vi "Begin.vi"(11 "Image Size":T1=enum."320x240") -> (0 "error out":errorcluster)   [LabVIEW 2012]
doc: "Called before other user functions, this VI is expected to open initial I/O refnums, load in file data, and do all program initialization. Notice that the <B>error out</B> terminal is simply used for data flow. Wiring it to other structures or subVIs ensures that this VI runs first."
uses:
  <vilib>/Rock Robotics/WPI/Camera/WPI_CameraImageSize.ctl
  <vilib>/Rock Robotics/WPI/Camera/WPI_CameraWhite Balance Values.ctl
  <vilib>/Rock Robotics/WPI/Camera/WPI_CameraExposure Values.ctl
  <vilib>/Rock Robotics/WPI/Camera/WPI_CameraFrameRate.ctl
  <vilib>/Rock Robotics/WPI/DriverStation/WPI_DriverStationRobotMode2.ctl
  <vilib>/Rock Robotics/WPI/Joystick/WPI_JoystickDeviceEnum.ctl
  <vilib>/Rock Robotics/WPI/CAN/Jaguar/SubVIs/WPI_CANJaguar_ControlMode.ctl
  <vilib>/Rock Robotics/WPI/CAN/Jaguar/SubVIs/WPI_CANJaguar_PositionReference.ctl
  <vilib>/Rock Robotics/WPI/CAN/Jaguar/SubVIs/WPI_CANJaguar_SpeedReference.ctl
  <vilib>/Rock Robotics/SystemInterfaces/Typedef/FPGA_TypedefDigitalModule.ctl
  <vilib>/Rock Robotics/SystemInterfaces/DIO/FPGA_DIOPWMChannel.ctl
  <vilib>/Rock Robotics/SystemInterfaces/DIO/FPGA_DIOChannel.ctl
  <vilib>/Rock Robotics/SystemInterfaces/DIO/FPGA_DIORelayChannel.ctl
  <vilib>/Rock Robotics/WPI/Relay/WPI_RelayDirection.ctl
  Robot Global Data.vi
  <vilib>/Rock Robotics/WPI/MotorControl/WPI_MotorControlOpenCANJaguar.vi
  <vilib>/Rock Robotics/WPI/MotorControl/WPI_MotorControlOpen Victor.vi
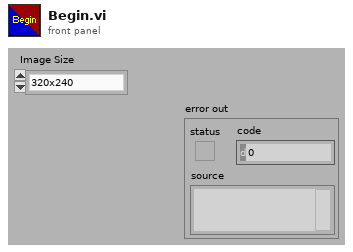
[diagram p1: front panel]
types:
  T1 = typedef "WPI_CameraImageSize.ctl" = enum16{"640x480", "320x240", "160x120"}
  T2 = typedef "WPI_RelayDirection.ctl" = enum16{"Both directions", "Forward only", "Reverse only"}
  T3 = typedef "FPGA_DIORelayChannel.ctl" = enum8{"Relay 1", "Relay 2", "Relay 3", "Relay 4", "Relay 5", "Relay 6", "Relay 7", "Relay 8", "Invalid"}
  T4 = typedef "FPGA_DIOChannel.ctl" = enum8{"DIO 1", "DIO 2", "DIO 3", "DIO 4", "DIO 5", "DIO 6", "DIO 7", "DIO 8", "DIO 9", "DIO 10", "DIO 11", "DIO 12", "DIO 13", "DIO 14", "Invalid"}
  T5 = typedef "FPGA_DIOPWMChannel.ctl" = enum8{"PWM 1", "PWM 2", "PWM 3", "PWM 4", "PWM 5", "PWM 6", "PWM 7", "PWM 8", "PWM 9", "PWM 10", "Invalid"}
  T6 = typedef "FPGA_TypedefDigitalModule.ctl" = enum16{"Digital Module 1", "Digital Module 2"}
  T7 = typedef "WPI_CANJaguar_SpeedReference.ctl" = u8
  T8 = typedef "WPI_CANJaguar_ControlMode.ctl" = enum8{"Percent VBus", "Current", "Speed", "Position", "Voltage"}
  T9 = typedef "WPI_CANJaguar_PositionReference.ctl" = u8
  T10 = typedef "WPI_JoystickDeviceEnum.ctl" = enum16{"USB 1", "USB 2", "USB 3", "USB 4", "Kinect 1", "Kinect 2"}
  T11 = typedef "WPI_DriverStationRobotMode2.ctl" = enum16{"Autonomous Disabled", "Autonomous Enabled", "Teleop Disabled", "Teleop Enabled", "Timeout", "Finish", "Test Disabled", "Test Enabled"}
  T12 = typedef "WPI_CameraFrameRate.ctl" = u32
  T13 = typedef "WPI_CameraExposure Values.ctl" = enum16{"Auto", "Flicker-free 50 Hz", "Flicker-free 60 Hz", "Hold current"}
  T14 = typedef "WPI_CameraWhite Balance Values.ctl" = enum16{"Auto", "Fixed indoor", "Fixed outdoor 1", "Fixed outdoor 2", "Fixed fluorescent 1", "Fixed fluorescent 2", "Hold current"}
  T15 = typedef "WPI_JoystickDevRef.ctl" = cluster{"Device":T10}
  T16 = typedef "WPI_CameraDevRef.ctl" = cluster{"Camera Address":string, "CameraStatus":errorcluster, "Acquire Image Notifier":refnum<notifier>}
  T17 = typedef "WPI_MotorControlDeviceRef.ctl" = cluster{"DeviceStatus":errorcluster, "Type":enum16{"PWM", "CAN"}, "PWM":cluster{"Digital Module":T6, "PWM Channel":T5, "DeadBand":T18}, "CAN":cluster{"Device Number":u8, "Control Mode":T8, "Semaphore":T19, "Max Vout":dbl}, "Invert":bool, "TransformRef":T20, "InvTransformRef":T20}
  T18 = typedef "WPI_PWMDeadband.ctl" = cluster{"Name":string, "maxPositivePwm":i32, "minPositivePwm":i32, "centerPwm":i32, "maxNegativePwm":i32, "minNegativePwm":i32, "angularRange":u16}
  T19 = typedef "Semaphore RefNum" = refnum<k1>
  T20 = typedef "WPI_PWMTransform_ConPane.ctl" = refnum<vi>
  T21 = typedef "WPI_DigitalInputDevRef.ctl" = cluster{"DevStatus":errorcluster, "DIO Channel":T4, "Digital Module":T6}
  T22 = typedef "WPI_RelayDevRef.ctl" = cluster{"DevStatus":errorcluster, "Relay Channel":T3, "Digital Module":T6, "Relay Direction":T2}
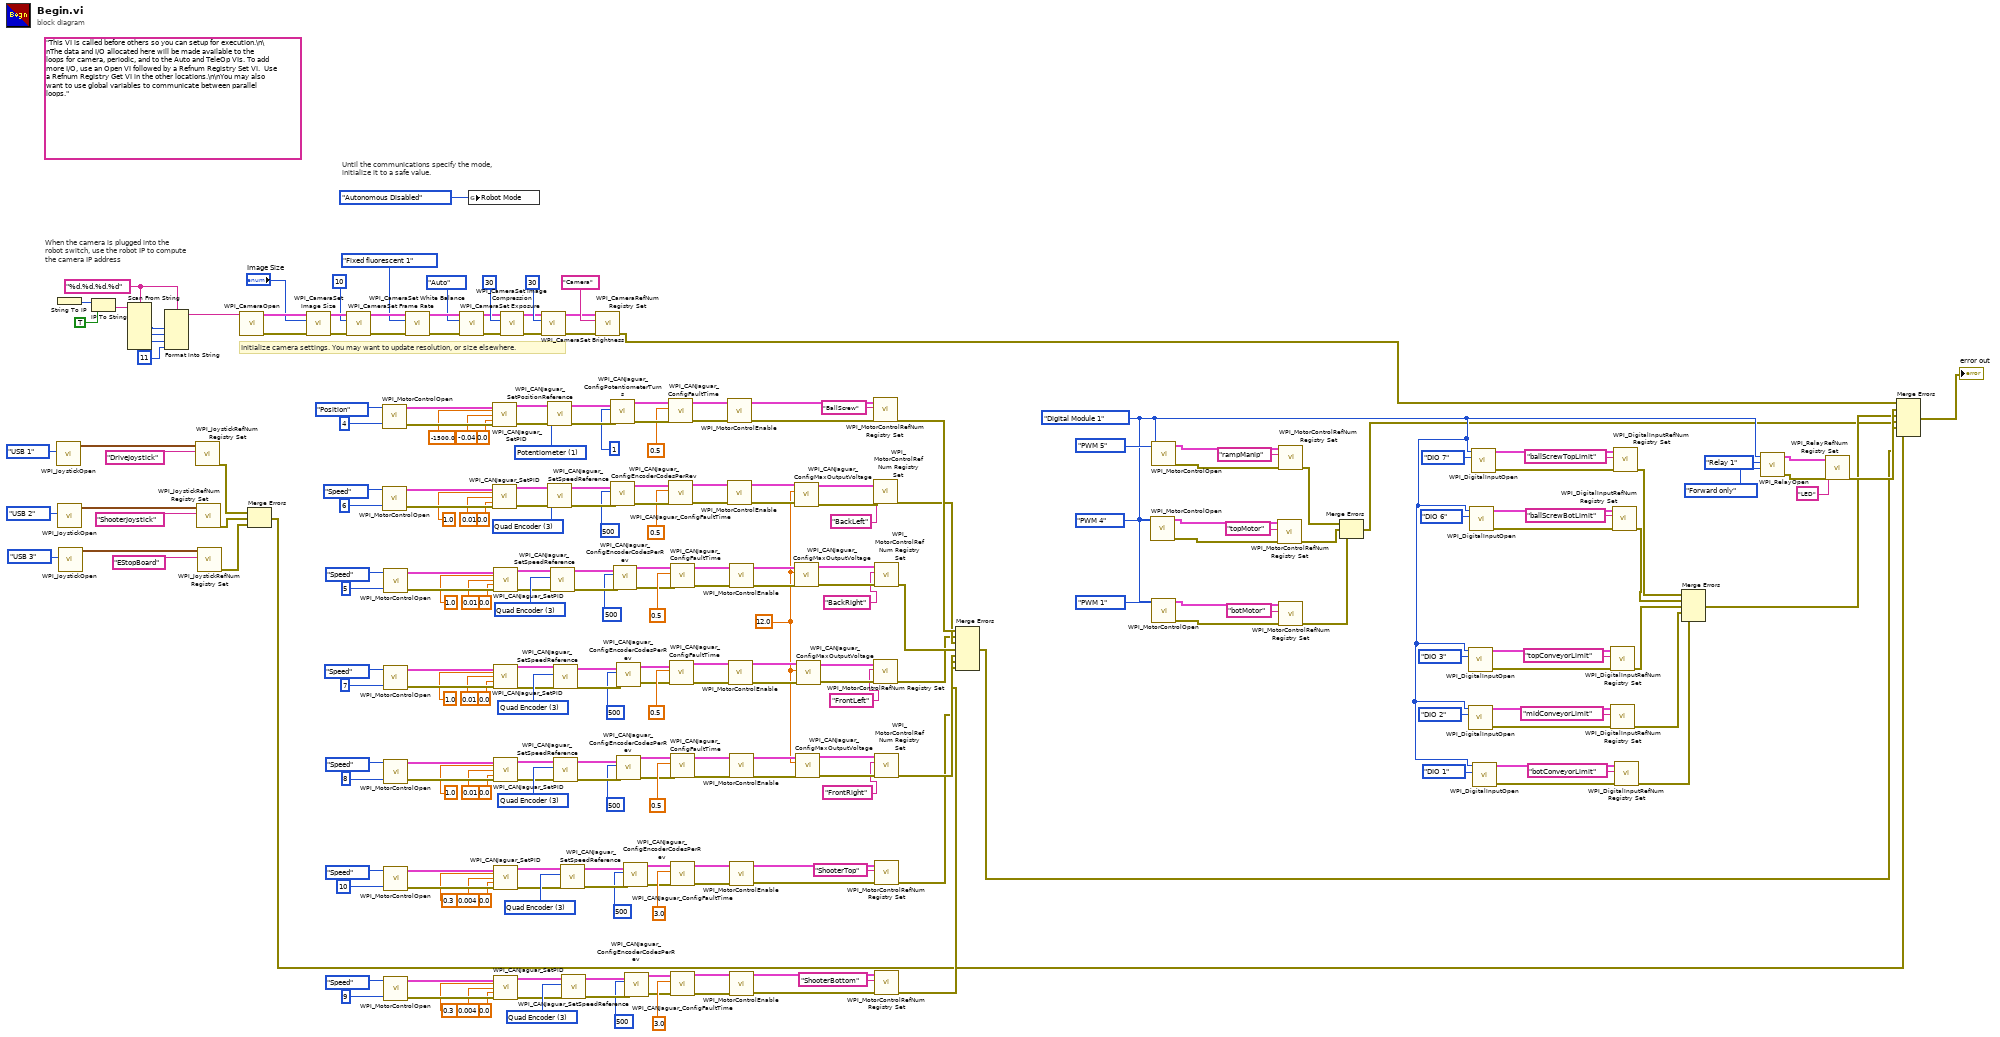
[diagram p0: block diagram]
diagram:
  w11 = FPGA_TypedefDigitalModule."Digital Module 1" ("Digital Module (Module 1)")
  w86 = T7 3 items=["Encoder"=0, "Inv Encoder"=2, "Quad Encoder"=3, "None"=255] ("Speed Reference")
  w90 = T7 3 items=["Encoder"=0, "Inv Encoder"=2, "Quad Encoder"=3, "None"=255] ("Speed Reference")
  w94 = T7 3 items=["Encoder"=0, "Inv Encoder"=2, "Quad Encoder"=3, "None"=255] ("Speed Reference")
  w98 = T7 3 items=["Encoder"=0, "Inv Encoder"=2, "Quad Encoder"=3, "None"=255] ("Speed Reference")
  w102 = T7 3 items=["Encoder"=0, "Inv Encoder"=2, "Quad Encoder"=3, "None"=255] ("Speed Reference")
  w106 = 12.0 ("Fault Time (s)")
  w127 = T7 3 items=["Encoder"=0, "Inv Encoder"=2, "Quad Encoder"=3, "None"=255] ("Speed Reference")
  w210 = T9 1 items=["Quad Encoder"=0, "Potentiometer"=1, "None"=255] ("Position Reference")
  w231 = "%d.%d.%d.%d" ("format string")
  (unwired) "This VI is called before others so you can setup for execution.\n\nThe data and I/O allocated here will be made available to the loops for camera, periodic, and to the Auto and TeleOp VIs. To add more I/O, use an Open VI followed by a Refnum Registry Set VI.  Use a Refnum Registry Get VI in the other locations.\n\nYou may also want to use global variables to communicate between parallel loops."
  # "Until the communications specify the mode,\ninitialize it to a safe value."
  # "When the camera is plugged into the\nrobot switch, use the robot IP to compute\nthe camera IP address"
  # "Initialize camera settings. You may want to update resolution, or size elsewhere."
  n1 = call <vilib>:"WPI_JoystickOpen.vi"("JoystickDevice"=WPI_JoystickDeviceEnum."USB 1") -> ("JoystickDevRef"=w227:T15)  [unwired: 10 in]
  n2 = String To IP() -> (0:w238:u32)  [unwired: 1 in]
  n3 = call <vilib>:"WPI_JoystickOpen.vi"("JoystickDevice"=WPI_JoystickDeviceEnum."USB 2") -> ("JoystickDevRef"=w224:T15)  [unwired: 10 in]
  n4 = call <vilib>:"WPI_JoystickOpen.vi"("JoystickDevice"=WPI_JoystickDeviceEnum."USB 3") -> ("JoystickDevRef"=w221:T15)  [unwired: 10 in]
  n5 = IP To String(1:TRUE ("dot notation? (F)"), 2:w238) -> (0:w236:string)
  n6 = Scan From String(format string=w231, input string=w236) -> (output 1=w235:i32, output 2=w234:i32, output 3=w233:i32)  [unwired: 7 in, 3 out]
  n7 = Format Into String(format string=w231, w235, w234, w233, 11 ("Compression")) -> (resulting string=w229:string)  [unwired: 2 in, 1 out]
  n8 = call <vilib>:"WPI_JoystickRefNum Registry Set.vi"("refnum name"="DriveJoystick", "JoystickDevRef"=w227) -> ("error out"=w63:errorcluster)  [unwired: 8 in, 1 out]
  n9 = call <vilib>:"WPI_JoystickRefNum Registry Set.vi"("refnum name"="ShooterJoystick", "JoystickDevRef"=w224) -> ("error out"=w62:errorcluster)  [unwired: 8 in, 1 out]
  n10 = call <vilib>:"WPI_JoystickRefNum Registry Set.vi"("refnum name"="EStopBoard", "JoystickDevRef"=w221) -> ("error out"=w61:errorcluster)  [unwired: 8 in, 1 out]
  n11 = call <vilib>:"WPI_CameraOpen.vi"("Camera Address"=w229) -> ("error out"=w250:errorcluster, "CameraDevRef"=w251:T16)  [unwired: 1 in, 8 out]
  n12 = Merge Errors(w63, w62, w61) -> (w2:errorcluster)
  n13 = call <vilib>:"WPI_CameraSet Image Size.vi"("error in (no error)"=w250, "Image Size"="Image Size", "CameraDevRef"=w251) -> ("error out"=w249:errorcluster, "CameraDevRef Out"=w252:T16)  [unwired: 7 out]
  n14 = call <vilib>:"WPI_CameraSet Frame Rate.vi"("error in (no error)"=w249, "Frame Rate (fps)"=T12 10, "CameraDevRef"=w252) -> ("error out"=w248:errorcluster, "CameraDevRef Out"=w254:T16)  [unwired: 7 out]
  n15 = call-poly <vilib>:"WPI_MotorControlOpen.vi"("Device Number"=u8 4, "Control Mode"=WPI_CANJaguar_ControlMode."Position") -> ("error out"=w216:errorcluster, "MotorControlDeviceRef"=w217:T17)  [unwired: 8 in]
  n16 = call-poly <vilib>:"WPI_MotorControlOpen.vi"("Device Number"=u8 6, "Control Mode"=WPI_CANJaguar_ControlMode."Speed") -> ("error out"=w196:errorcluster, "MotorControlDeviceRef"=w197:T17)  [unwired: 8 in]
  n17 = call-poly <vilib>:"WPI_MotorControlOpen.vi"("Device Number"=u8 7, "Control Mode"=WPI_CANJaguar_ControlMode."Speed") -> ("error out"=w169:errorcluster, "MotorControlDeviceRef"=w170:T17)  [unwired: 8 in]
  n18 = call-poly <vilib>:"WPI_MotorControlOpen.vi"("Device Number"=u8 5, "Control Mode"=WPI_CANJaguar_ControlMode."Speed") -> ("error out"=w179:errorcluster, "MotorControlDeviceRef"=w180:T17)  [unwired: 8 in]
  n19 = call-poly <vilib>:"WPI_MotorControlOpen.vi"("Device Number"=u8 8, "Control Mode"=WPI_CANJaguar_ControlMode."Speed") -> ("error out"=w159:errorcluster, "MotorControlDeviceRef"=w160:T17)  [unwired: 8 in]
  n20 = call-poly <vilib>:"WPI_MotorControlOpen.vi"("Device Number"=u8 10, "Control Mode"=WPI_CANJaguar_ControlMode."Speed") -> ("error out"=w149:errorcluster, "MotorControlDeviceRef"=w150:T17)  [unwired: 8 in]
  n21 = call-poly <vilib>:"WPI_MotorControlOpen.vi"("Device Number"=u8 9, "Control Mode"=WPI_CANJaguar_ControlMode."Speed") -> ("error out"=w137:errorcluster, "MotorControlDeviceRef"=w138:T17)  [unwired: 8 in]
  n22 = call <vilib>:"WPI_CameraSet White Balance.vi"("error in (no error)"=w248, "White Balance"=WPI_CameraWhite_Balance_Values."Fixed fluorescent 1", "CameraDevRef"=w254) -> ("error out"=w247:errorcluster, "CameraDevRef Out"=w253:T16)  [unwired: 7 out]
  n23 = call <vilib>:"WPI_CameraSet Exposure.vi"("error in (no error)"=w247, "Exposure"=WPI_CameraExposure_Values."Auto", "CameraDevRef"=w253) -> ("error out"=w246:errorcluster, "CameraDevRef Out"=w256:T16)  [unwired: 7 out]
  n24 = global write "Robot Global Data.vi" "Robot Mode"(WPI_DriverStationRobotMode2."Autonomous Disabled" ("Robot Mode")) -> ()
  n25 = call <vilib>:"WPI_CANJaguar_SetPID.vi"("CAN Jaguar Ref"=w217, "P"=-1500.0, "I"=-0.04, "D"=0.0, "error in (no error)"=w216) -> ("CAN Jaguar Ref Out"=w212:T17, "error out"=w211:errorcluster)  [unwired: 9 in]
  n26 = call <vilib>:"WPI_CANJaguar_SetPID.vi"("CAN Jaguar Ref"=w197, "P"=1.0, "I"=0.01, "D"=0.0, "error in (no error)"=w196) -> ("CAN Jaguar Ref Out"=w192:T17, "error out"=w191:errorcluster)  [unwired: 9 in]
  n27 = call <vilib>:"WPI_CANJaguar_SetPID.vi"("CAN Jaguar Ref"=w170, "P"=1.0, "I"=0.01, "D"=0.0, "error in (no error)"=w169) -> ("CAN Jaguar Ref Out"=w69:T17, "error out"=w68:errorcluster)  [unwired: 9 in]
  n28 = call <vilib>:"WPI_CANJaguar_SetPID.vi"("CAN Jaguar Ref"=w180, "P"=1.0, "I"=0.01, "D"=0.0, "error in (no error)"=w179) -> ("CAN Jaguar Ref Out"=w73:T17, "error out"=w72:errorcluster)  [unwired: 9 in]
  n29 = call <vilib>:"WPI_CANJaguar_SetPID.vi"("CAN Jaguar Ref"=w160, "P"=1.0, "I"=0.01, "D"=0.0, "error in (no error)"=w159) -> ("CAN Jaguar Ref Out"=w76:T17, "error out"=w77:errorcluster)  [unwired: 9 in]
  n30 = call <vilib>:"WPI_CANJaguar_SetPID.vi"("CAN Jaguar Ref"=w150, "P"=0.3, "I"=0.004, "D"=0.0, "error in (no error)"=w149) -> ("CAN Jaguar Ref Out"=w78:T17, "error out"=w79:errorcluster)  [unwired: 9 in]
  n31 = call <vilib>:"WPI_CANJaguar_SetPID.vi"("CAN Jaguar Ref"=w138, "P"=0.3, "I"=0.004, "D"=0.0, "error in (no error)"=w137) -> ("CAN Jaguar Ref Out"=w85:T17, "error out"=w84:errorcluster)  [unwired: 9 in]
  n32 = call <vilib>:"WPI_CameraSet Image Compression.vi"("error in (no error)"=w246, "Compression"=30, "CameraDevRef"=w256) -> ("error out"=w245:errorcluster, "CameraDevRef Out"=w255:T16)  [unwired: 7 out]
  n33 = call <vilib>:"WPI_CameraSet Brightness.vi"("error in (no error)"=w245, "Brightness"=30, "CameraDevRef"=w255) -> ("error out"=w243:errorcluster, "CameraDevRef Out"=w244:T16)  [unwired: 7 out]
  n34 = call <vilib>:"WPI_CANJaguar_SetPositionReference.vi"("error in (no error)"=w211, "Position Reference"=w210, "CAN Jaguar Ref"=w212) -> ("error out"=w208:errorcluster, "CAN Jaguar Ref Out"=w209:T17)  [unwired: 7 in]
  n35 = call <vilib>:"WPI_CANJaguar_SetSpeedReference.vi"("error in (no error)"=w191, "Speed Reference"=w127, "CAN Jaguar Ref"=w192) -> ("error out"=w189:errorcluster, "CAN Jaguar Ref Out"=w190:T17)  [unwired: 7 in]
  n36 = call <vilib>:"WPI_CANJaguar_SetSpeedReference.vi"("error in (no error)"=w72, "Speed Reference"=w102, "CAN Jaguar Ref"=w73) -> ("error out"=w104:errorcluster, "CAN Jaguar Ref Out"=w105:T17)  [unwired: 7 in]
  n37 = call <vilib>:"WPI_CANJaguar_SetSpeedReference.vi"("error in (no error)"=w68, "Speed Reference"=w98, "CAN Jaguar Ref"=w69) -> ("error out"=w100:errorcluster, "CAN Jaguar Ref Out"=w101:T17)  [unwired: 7 in]
  n38 = call <vilib>:"WPI_CANJaguar_SetSpeedReference.vi"("error in (no error)"=w77, "Speed Reference"=w94, "CAN Jaguar Ref"=w76) -> ("error out"=w96:errorcluster, "CAN Jaguar Ref Out"=w97:T17)  [unwired: 7 in]
  n39 = call <vilib>:"WPI_CANJaguar_SetSpeedReference.vi"("error in (no error)"=w79, "Speed Reference"=w90, "CAN Jaguar Ref"=w78) -> ("error out"=w92:errorcluster, "CAN Jaguar Ref Out"=w93:T17)  [unwired: 7 in]
  n40 = call <vilib>:"WPI_CANJaguar_SetSpeedReference.vi"("error in (no error)"=w84, "Speed Reference"=w86, "CAN Jaguar Ref"=w85) -> ("error out"=w88:errorcluster, "CAN Jaguar Ref Out"=w89:T17)  [unwired: 7 in]
  n41 = call <vilib>:"WPI_CameraRefNum Registry Set.vi"("error in (no error)"=w243, "refnum name"="Camera", "CameraDevRef"=w244) -> ("error out"=w1:errorcluster)  [unwired: 8 out]
  n42 = call <vilib>:"WPI_CANJaguar_ConfigPotentiometerTurns.vi"("error in (no error)"=w208, "Potentiometer Turns"=u16 1, "CAN Jaguar Ref"=w209) -> ("error out"=w205:errorcluster, "CAN Jaguar Ref Out"=w206:T17)  [unwired: 7 in]
  n43 = call <vilib>:"WPI_CANJaguar_ConfigEncoderCodesPerRev.vi"("error in (no error)"=w189, "Encoder Codes Per Rev"=u16 500 ("Potentiometer Turns"), "CAN Jaguar Ref"=w190) -> ("error out"=w186:errorcluster, "CAN Jaguar Ref Out"=w187:T17)  [unwired: 7 in]
  n44 = call <vilib>:"WPI_CANJaguar_ConfigEncoderCodesPerRev.vi"("error in (no error)"=w104, "Encoder Codes Per Rev"=u16 500 ("Potentiometer Turns"), "CAN Jaguar Ref"=w105) -> ("error out"=w71:errorcluster, "CAN Jaguar Ref Out"=w70:T17)  [unwired: 7 in]
  n45 = call <vilib>:"WPI_CANJaguar_ConfigEncoderCodesPerRev.vi"("error in (no error)"=w100, "Encoder Codes Per Rev"=u16 500 ("Potentiometer Turns"), "CAN Jaguar Ref"=w101) -> ("error out"=w66:errorcluster, "CAN Jaguar Ref Out"=w67:T17)  [unwired: 7 in]
  n46 = call <vilib>:"WPI_CANJaguar_ConfigEncoderCodesPerRev.vi"("error in (no error)"=w96, "Encoder Codes Per Rev"=u16 500 ("Potentiometer Turns"), "CAN Jaguar Ref"=w97) -> ("error out"=w75:errorcluster, "CAN Jaguar Ref Out"=w74:T17)  [unwired: 7 in]
  n47 = call <vilib>:"WPI_CANJaguar_ConfigEncoderCodesPerRev.vi"("error in (no error)"=w92, "Encoder Codes Per Rev"=u16 500 ("Potentiometer Turns"), "CAN Jaguar Ref"=w93) -> ("error out"=w81:errorcluster, "CAN Jaguar Ref Out"=w80:T17)  [unwired: 7 in]
  n48 = call <vilib>:"WPI_CANJaguar_ConfigEncoderCodesPerRev.vi"("error in (no error)"=w88, "Encoder Codes Per Rev"=u16 500 ("Potentiometer Turns"), "CAN Jaguar Ref"=w89) -> ("error out"=w82:errorcluster, "CAN Jaguar Ref Out"=w83:T17)  [unwired: 7 in]
  n49 = call <vilib>:"WPI_CANJaguar_ConfigFaultTime.vi"("error in (no error)"=w205, "Fault Time (s)"=0.5, "CAN Jaguar Ref"=w206) -> ("error out"=w202:errorcluster, "CAN Jaguar Ref Out"=w203:T17)  [unwired: 7 in]
  n50 = call <vilib>:"WPI_CANJaguar_ConfigFaultTime.vi"("error in (no error)"=w186, "Fault Time (s)"=0.5, "CAN Jaguar Ref"=w187) -> ("error out"=w183:errorcluster, "CAN Jaguar Ref Out"=w184:T17)  [unwired: 7 in]
  n51 = call <vilib>:"WPI_CANJaguar_ConfigFaultTime.vi"("error in (no error)"=w66, "Fault Time (s)"=0.5, "CAN Jaguar Ref"=w67) -> ("error out"=w163:errorcluster, "CAN Jaguar Ref Out"=w164:T17)  [unwired: 7 in]
  n52 = call <vilib>:"WPI_CANJaguar_ConfigFaultTime.vi"("error in (no error)"=w71, "Fault Time (s)"=0.5, "CAN Jaguar Ref"=w70) -> ("error out"=w173:errorcluster, "CAN Jaguar Ref Out"=w174:T17)  [unwired: 7 in]
  n53 = call <vilib>:"WPI_CANJaguar_ConfigFaultTime.vi"("error in (no error)"=w75, "Fault Time (s)"=0.5, "CAN Jaguar Ref"=w74) -> ("error out"=w153:errorcluster, "CAN Jaguar Ref Out"=w154:T17)  [unwired: 7 in]
  n54 = call <vilib>:"WPI_CANJaguar_ConfigFaultTime.vi"("error in (no error)"=w81, "Fault Time (s)"=3.0, "CAN Jaguar Ref"=w80) -> ("error out"=w143:errorcluster, "CAN Jaguar Ref Out"=w144:T17)  [unwired: 7 in]
  n55 = call <vilib>:"WPI_CANJaguar_ConfigFaultTime.vi"("error in (no error)"=w82, "Fault Time (s)"=3.0, "CAN Jaguar Ref"=w83) -> ("error out"=w131:errorcluster, "CAN Jaguar Ref Out"=w132:T17)  [unwired: 7 in]
  n56 = call <vilib>:"WPI_MotorControlEnable.vi"("error in (no error)"=w202, "CAN Jaguar Ref"=w203) -> ("error out"=w200:errorcluster, "CAN Jaguar Ref Out"=w201:T17)  [unwired: 8 in]
  n57 = call <vilib>:"WPI_MotorControlEnable.vi"("error in (no error)"=w183, "CAN Jaguar Ref"=w184) -> ("error out"=w125:errorcluster, "CAN Jaguar Ref Out"=w126:T17)  [unwired: 8 in]
  n58 = call <vilib>:"WPI_MotorControlEnable.vi"("error in (no error)"=w163, "CAN Jaguar Ref"=w164) -> ("error out"=w113:errorcluster, "CAN Jaguar Ref Out"=w114:T17)  [unwired: 8 in]
  n59 = call <vilib>:"WPI_MotorControlEnable.vi"("error in (no error)"=w173, "CAN Jaguar Ref"=w174) -> ("error out"=w120:errorcluster, "CAN Jaguar Ref Out"=w121:T17)  [unwired: 8 in]
  n60 = call <vilib>:"WPI_MotorControlEnable.vi"("error in (no error)"=w153, "CAN Jaguar Ref"=w154) -> ("error out"=w110:errorcluster, "CAN Jaguar Ref Out"=w111:T17)  [unwired: 8 in]
  n61 = call <vilib>:"WPI_MotorControlEnable.vi"("error in (no error)"=w143, "CAN Jaguar Ref"=w144) -> ("error out"=w141:errorcluster, "CAN Jaguar Ref Out"=w142:T17)  [unwired: 8 in]
  n62 = call <vilib>:"WPI_MotorControlEnable.vi"("error in (no error)"=w131, "CAN Jaguar Ref"=w132) -> ("error out"=w129:errorcluster, "CAN Jaguar Ref Out"=w130:T17)  [unwired: 8 in]
  n63 = call <vilib>:"WPI_CANJaguar_ConfigMaxOutputVoltage.vi"("error in (no error)"=w120, "Maximum Output Voltage"=w106, "CAN Jaguar Ref"=w121) -> ("error out"=w119:errorcluster, "CAN Jaguar Ref Out"=w118:T17)  [unwired: 7 in]
  n64 = call <vilib>:"WPI_CANJaguar_ConfigMaxOutputVoltage.vi"("error in (no error)"=w125, "Maximum Output Voltage"=w106, "CAN Jaguar Ref"=w126) -> ("error out"=w124:errorcluster, "CAN Jaguar Ref Out"=w123:T17)  [unwired: 7 in]
  n65 = call <vilib>:"WPI_CANJaguar_ConfigMaxOutputVoltage.vi"("error in (no error)"=w110, "Maximum Output Voltage"=w106, "CAN Jaguar Ref"=w111) -> ("error out"=w108:errorcluster, "CAN Jaguar Ref Out"=w109:T17)  [unwired: 7 in]
  n66 = call <vilib>:"WPI_CANJaguar_ConfigMaxOutputVoltage.vi"("error in (no error)"=w113, "Maximum Output Voltage"=w106, "CAN Jaguar Ref"=w114) -> ("error out"=w115:errorcluster, "CAN Jaguar Ref Out"=w116:T17)  [unwired: 7 in]
  n67 = call <vilib>:"WPI_MotorControlRefNum Registry Set.vi"("error in (no error)"=w200, "refnum name"="BallScrew", "MotorControlDevRef"=w201) -> ("error out"=w60:errorcluster)  [unwired: 7 in, 1 out]
  n68 = call <vilib>:"WPI_MotorControlRefNum Registry Set.vi"("error in (no error)"=w124, "refnum name"="BackLeft", "MotorControlDevRef"=w123) -> ("error out"=w59:errorcluster)  [unwired: 7 in, 1 out]
  n69 = call <vilib>:"WPI_MotorControlRefNum Registry Set.vi"("error in (no error)"=w115, "refnum name"="FrontLeft", "MotorControlDevRef"=w116) -> ("error out"=w57:errorcluster)  [unwired: 7 in, 1 out]
  n70 = call <vilib>:"WPI_MotorControlRefNum Registry Set.vi"("error in (no error)"=w119, "refnum name"="BackRight", "MotorControlDevRef"=w118) -> ("error out"=w58:errorcluster)  [unwired: 7 in, 1 out]
  n71 = call <vilib>:"WPI_MotorControlRefNum Registry Set.vi"("error in (no error)"=w108, "refnum name"="FrontRight", "MotorControlDevRef"=w109) -> ("error out"=w56:errorcluster)  [unwired: 7 in, 1 out]
  n72 = call <vilib>:"WPI_MotorControlRefNum Registry Set.vi"("error in (no error)"=w141, "refnum name"="ShooterTop", "MotorControlDevRef"=w142) -> ("error out"=w55:errorcluster)  [unwired: 7 in, 1 out]
  n73 = call <vilib>:"WPI_MotorControlRefNum Registry Set.vi"("error in (no error)"=w129, "refnum name"="ShooterBottom", "MotorControlDevRef"=w130) -> ("error out"=w54:errorcluster)  [unwired: 7 in, 1 out]
  n74 = Merge Errors(w60, w57, w59, w58, w56, w55, w54) -> (w3:errorcluster)
  n75 = call-poly <vilib>:"WPI_MotorControlOpen.vi"("PWM Channel"=FPGA_DIOPWMChannel."PWM 4", "Digital Module (Module 1)"=w11) -> ("error out"=w46:errorcluster, "MotorControlDeviceRef"=w48:T17)  [unwired: 8 in]
  n76 = call-poly <vilib>:"WPI_MotorControlOpen.vi"("PWM Channel"=FPGA_DIOPWMChannel."PWM 5", "Digital Module (Module 1)"=w11) -> ("error out"=w50:errorcluster, "MotorControlDeviceRef"=w52:T17)  [unwired: 8 in]
  n77 = call-poly <vilib>:"WPI_MotorControlOpen.vi"("PWM Channel"=FPGA_DIOPWMChannel."PWM 1", "Digital Module (Module 1)"=w11) -> ("error out"=w42:errorcluster, "MotorControlDeviceRef"=w44:T17)  [unwired: 8 in]
  n78 = call <vilib>:"WPI_MotorControlRefNum Registry Set.vi"("error in (no error)"=w46, "refnum name"="topMotor", "MotorControlDevRef"=w48) -> ("error out"=w40:errorcluster)  [unwired: 7 in, 1 out]
  n79 = call <vilib>:"WPI_MotorControlRefNum Registry Set.vi"("error in (no error)"=w50, "refnum name"="rampManip", "MotorControlDevRef"=w52) -> ("error out"=w41:errorcluster)  [unwired: 7 in, 1 out]
  n80 = call <vilib>:"WPI_MotorControlRefNum Registry Set.vi"("error in (no error)"=w42, "refnum name"="botMotor", "MotorControlDevRef"=w44) -> ("error out"=w39:errorcluster)  [unwired: 7 in, 1 out]
  n81 = Merge Errors(w41, w40, w39) -> (w4:errorcluster)
  n82 = call <vilib>:"WPI_DigitalInputOpen.vi"("DIO Channel"=FPGA_DIOChannel."DIO 3", "Digital Module (Module 1)"=w11) -> ("error out"=w28:errorcluster, "DigitalInputDevRef"=w29:T21)  [unwired: 8 in]
  n83 = call <vilib>:"WPI_DigitalInputOpen.vi"("DIO Channel"=FPGA_DIOChannel."DIO 2", "Digital Module (Module 1)"=w11) -> ("error out"=w24:errorcluster, "DigitalInputDevRef"=w25:T21)  [unwired: 8 in]
  n84 = call <vilib>:"WPI_DigitalInputOpen.vi"("DIO Channel"=FPGA_DIOChannel."DIO 6", "Digital Module (Module 1)"=w11) -> ("error out"=w32:errorcluster, "DigitalInputDevRef"=w33:T21)  [unwired: 8 in]
  n85 = call <vilib>:"WPI_DigitalInputOpen.vi"("DIO Channel"=FPGA_DIOChannel."DIO 7", "Digital Module (Module 1)"=w11) -> ("error out"=w36:errorcluster, "DigitalInputDevRef"=w37:T21)  [unwired: 8 in]
  n86 = call <vilib>:"WPI_DigitalInputOpen.vi"("DIO Channel"=FPGA_DIOChannel."DIO 1", "Digital Module (Module 1)"=w11) -> ("error out"=w20:errorcluster, "DigitalInputDevRef"=w21:T21)  [unwired: 8 in]
  n87 = call <vilib>:"WPI_DigitalInputRefNum Registry Set.vi"("error in (no error)"=w28, "refnum name"="topConveyorLimit", "DigitalInputDevRef"=w29) -> ("error out"=w16:errorcluster)  [unwired: 7 in, 1 out]
  n88 = call <vilib>:"WPI_DigitalInputRefNum Registry Set.vi"("error in (no error)"=w24, "refnum name"="midConveyorLimit", "DigitalInputDevRef"=w25) -> ("error out"=w15:errorcluster)  [unwired: 7 in, 1 out]
  n89 = call <vilib>:"WPI_DigitalInputRefNum Registry Set.vi"("error in (no error)"=w32, "refnum name"="ballScrewBotLimit", "DigitalInputDevRef"=w33) -> ("error out"=w17:errorcluster)  [unwired: 7 in, 1 out]
  n90 = call <vilib>:"WPI_DigitalInputRefNum Registry Set.vi"("error in (no error)"=w36, "refnum name"="ballScrewTopLimit", "DigitalInputDevRef"=w37) -> ("error out"=w18:errorcluster)  [unwired: 7 in, 1 out]
  n91 = call <vilib>:"WPI_DigitalInputRefNum Registry Set.vi"("error in (no error)"=w20, "refnum name"="botConveyorLimit", "DigitalInputDevRef"=w21) -> ("error out"=w14:errorcluster)  [unwired: 7 in, 1 out]
  n92 = Merge Errors(w18, w17, w16, w15, w14) -> (w5:errorcluster)
  n93 = call <vilib>:"WPI_RelayOpen.vi"("Relay Direction"=WPI_RelayDirection."Forward only", "Relay Channel"=FPGA_DIORelayChannel."Relay 1", "Digital Module (Module 1)"=w11) -> ("error out"=w9:errorcluster, "RelayDevRef"=w8:T22)  [unwired: 7 in]
  n94 = call <vilib>:"WPI_RelayRefNum Registry Set.vi"("error in (no error)"=w9, "refnum name"="LED", "RelayDevRef"=w8) -> ("error out"=w6:errorcluster)  [unwired: 7 in, 1 out]
  n95 = Merge Errors(w1, w6, w5, w4, w3, w2) -> (→"error out":errorcluster)
